vi "Enable.vi"(8 "error in (no error)":errorcluster, 10 "Enable?":bool, 11 "Name":string) -> (0 "error out":errorcluster)   [LabVIEW 2017, in "TimerEngine.lvlib" / "TimerEngine.lvclass"]
uses:
  TimerEngine.lvclass
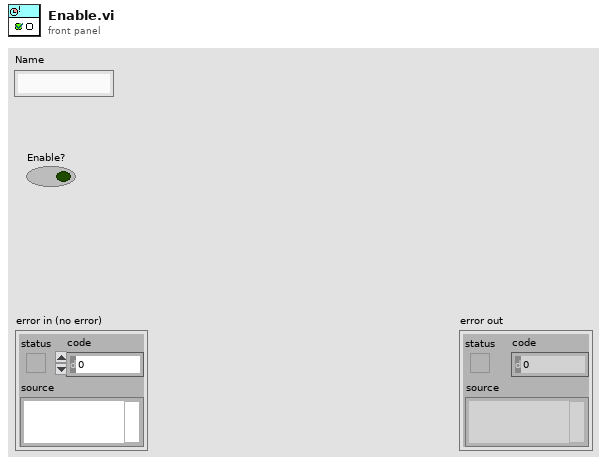
[diagram p1: front panel]
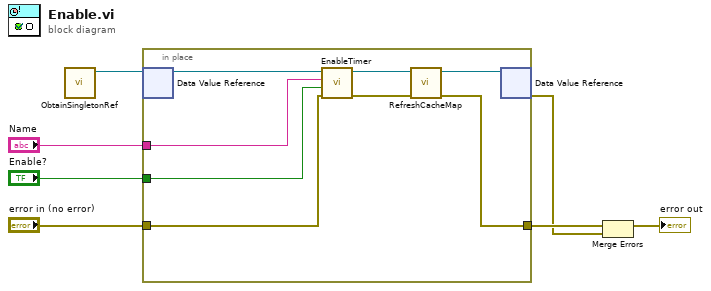
[diagram p0: block diagram]
diagram:
  n1 = call "ObtainSingletonRef.vi"() -> ("data value reference"=w7:refnum<data-value>)  [unwired: 10 in, 1 out]
  n2 = in-place {
    in-place-border: [w8] -> w6
    in-place-border: "error in (no error)" -> [w13]
    in-place-border: "Name" -> [w12]
    in-place-border: "Enable?" -> [w11]
    n3 = in-place-dvr #1(w7) -> (w15:refnum<class "TimerEngine.lvclass">)  [unwired: 1 out]
    n4 = call "EnableTimer.vi"("error in (no error)"=w13, "Enable?"=w11, "Name"=w12, "TimerEngine in"=w15) -> ("error out"=w9:errorcluster, "TimerEngine out"=w14:refnum<class "TimerEngine.lvclass">)  [unwired: 6 in]
    n5 = call "RefreshCacheMap.vi"("error in (no error)"=w9, "UserEventTimer in"=w14) -> ("error out"=w8:errorcluster, "UserEventTimer out"=w10:refnum<class "TimerEngine.lvclass">)  [unwired: 8 in]
    n6 = in-place-dvr #1(w10) -> (w3:errorcluster)  [unwired: 1 out]
  }
  n7 = Merge Errors(w6, w3) -> (→"error out":errorcluster)
